vi "FixHistogramSamplingvi.vi"(10 "Sampling Interval":dbl, 11 "Histogram in":T1(graph)) -> (3 "Histogram out":T1(graph))   [LabVIEW 2012]
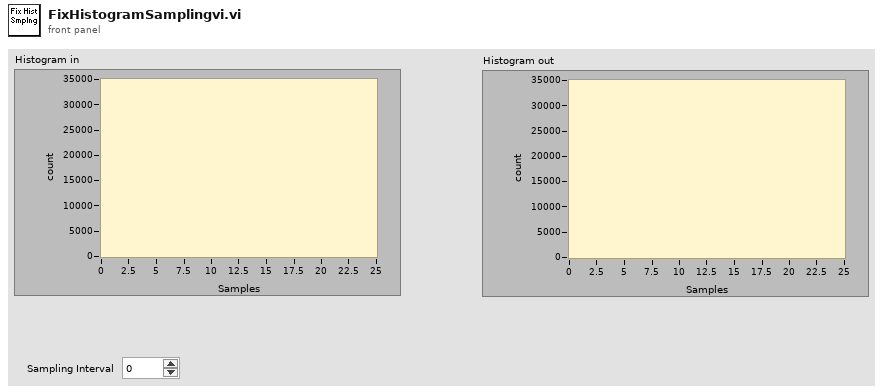
[diagram p1: front panel]
types:
  T1 = cluster{"X Values":dbl[], "Histogram: h(x)":i32[]}
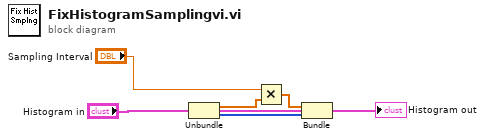
[diagram p0: block diagram]
diagram:
  n1 = Unbundle("Histogram in") -> ("X Values"=w3:dbl[], "Histogram: h(x)"=w4:i32[])
  n2 = Multiply(x="Sampling Interval", y=w3) -> (x*y=w2:dbl[])
  n3 = Bundle(cluster="Histogram in", "X Values"=w2, "Histogram: h(x)"=w4) -> (→"Histogram out":T1)
